vi "TRF to TSP Plot_05_15_13a_JW.vi"(8 "Transport Graph Properties":T1={"Transport Line Size"=0, "Transport Line Color"=16774656} {"Transport Line Size" items=["Extra Small", "Small", "Medium", "Large", "Extra Large"]}, 9 "No Transport File":path=path "\\\\acad1\\physics/Jurchescu-group/JW-PD/Mega Awesome/No Transport File.txt", 10 "Transport Folder":path, 11 "Transfer File":path) -> (1 "Transport":cluster{ext[], ext[]}[](graph), 2 "Transport File":path, 3 "Transport Name":string)   [LabVIEW 2015]
uses:
  <vilib>/Utility/file.llb/Read From Spreadsheet File (string).vi
  <vilib>/regexp/Match Regular Expression.xnode
panel:
  in  "default (0 dbl)":ext format="%.2e"
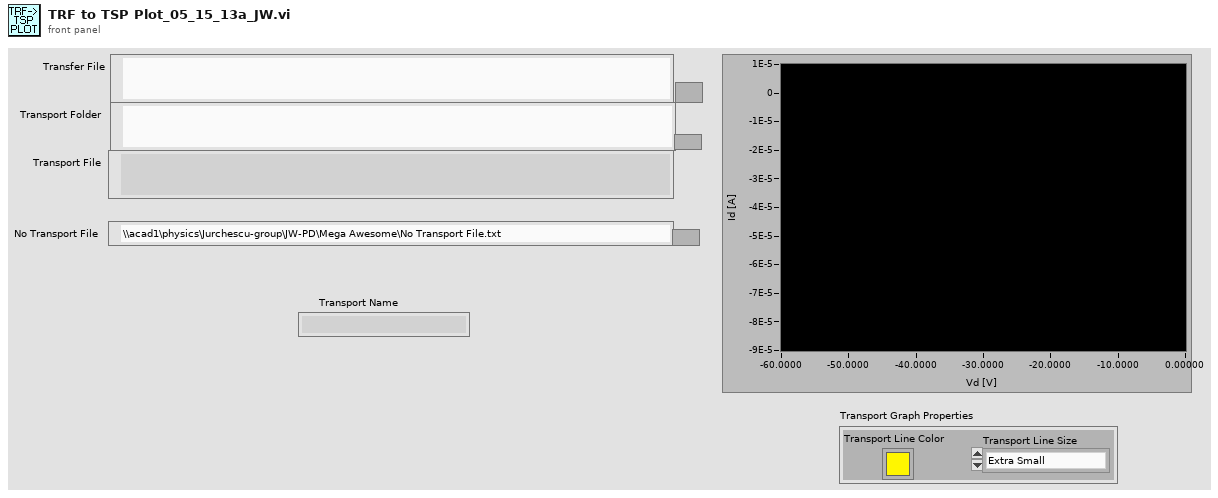
[diagram p1: front panel]
types:
  T1 = cluster{"Transport Line Size":u16, "Transport Line Color":u32}
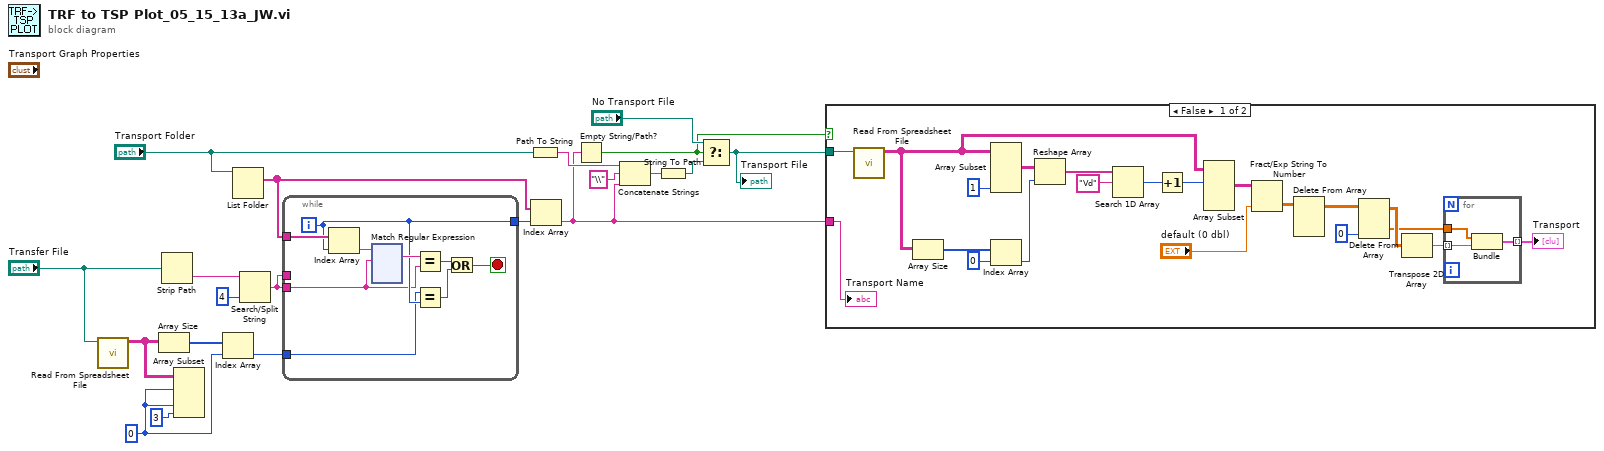
[diagram p0: block diagram]
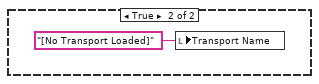
[diagram p2: hidden frame]
diagram:
  w20 = 0
  n1 = call-poly <vilib>:"Read From Spreadsheet File.vi"("file path (dialog if empty)"="Transfer File") -> ("all rows"=w17:string[][])  [unwired: 6 in, 4 out]
  n2 = Array Size(array=w17) -> (size(s)=w19:i32[])
  n3 = Strip Path(path="Transfer File") -> (name=w3:string)  [unwired: 1 out]
  n4 = Array Subset(array=w17, index (row)=w20, index (col)=w20, length (col)=3) -> ()  [unwired: 1 in, 1 out]
  n5 = Index Array(array=w19, index=w20) -> (element=w16:i32)
  n6 = List Folder(path="Transport Folder") -> (filenames=w13:string[])  [unwired: 3 in, 3 out]
  n7 = Search/Split String(string=w3, offset (0)=4) -> (match + rest of string=w1:string)  [unwired: 1 in, 2 out]
  n8 = while {
    tunnel: w13 -> [w28]
    tunnel: [w26] -> w14
    tunnel: w16 -> [w25]
    tunnel: w1 -> [_]
    tunnel: w1 -> [w21]
    i -> [w26]
    stop <- w22 stop-if-true
    n9 = Index Array(array=w28, index=w26) -> (element=w29:string)
    n10 = xnode "Match Regular Expression"("input string"=w29, "regular expression"=w21) -> ("whole match"=w27:string)  [unwired: 4 in, 4 out]
    n11 = Equal?(x=w27, y=w21) -> (x = y?=w24:bool)
    n12 = Equal?(x=w25, y=w26) -> (x = y?=w23:bool)
    n13 = Or(x=w24, y=w23) -> (x .or. y?=w22:bool)
  }
  n14 = Path To String(path="Transport Folder") -> (string=w10:string)
  n15 = Index Array(array=w13, index=w14) -> (element=w7:string)
  n16 = Empty String/Path?(string/path=w7) -> (empty?=w5:bool)
  n17 = Concatenate Strings(w10, "\\", w7) -> (w11:string)
  n18 = String To Path(string=w11) -> (path=w8:path)
  n19 = Select(t="No Transport File", s=w5, f=w8) -> (s? t:f=w9:path)
  "Transport File" <- w9
  n20 = case shown="False" w5 {
    tunnel: w9 -> [w161 _]
    tunnel: w7 -> [w141 _]
    frame False {
      n21 = call-poly <vilib>:"Read From Spreadsheet File.vi"("file path (dialog if empty)"=w161) -> ("all rows"=w154:string[][])  [unwired: 6 in, 4 out]
      n22 = Array Size(array=w154) -> (size(s)=w160:i32[])
      n23 = Array Subset(array=w154, length (col)=1) -> (w156:string[][])  [unwired: 3 in]
      n24 = Index Array(array=w160, index=0) -> (element=w149:i32)
      n25 = Reshape Array(w156, w149) -> (w155:string[])
      n26 = Search 1D Array(1D array=w155, element="Vd") -> (index of element=w153:i32)  [unwired: 1 in]
      n27 = Increment(x=w153) -> (x+1=w152:i32)
      n28 = Array Subset(array=w154, index (row)=w152) -> (w150:string[][])  [unwired: 3 in]
      n29 = Fract/Exp String To Number(string=w150, default (0 dbl)="default (0 dbl)") -> (number=w144:ext[][])  [unwired: 2 in, 1 out]
      n30 = Delete From Array(array=w144) -> (array with subset deleted=w143:ext[][])  [unwired: 3 in, 1 out]
      n31 = Delete From Array(array=w143, index (col)=0 ("Deaktivierter Index (Spalte)")) -> (deleted portion=w146:ext[], array with subset deleted=w147:ext[][])  [unwired: 2 in]
      n32 = Transpose 2D Array(2D array=w147) -> (transposed array=w148:ext[][])
      n33 = for {
        tunnel: w146 -> [w163]
        tunnel: w148 -> [w164] mode=indexing
        tunnel: [w162] -> w142 mode=indexing
        n34 = Bundle(w163, w164) -> (w162:cluster{ext[], ext[]})  [unwired: 1 in]
      }
      "Transport" <- w142
      "Transport Name" <- w141
    }
    frame True {
      n35 = local write "Transport Name"("[No Transport Loaded]") -> ()
    }
  }
